vi "Tester.vi"   [LabVIEW 2012]
uses:
  <vilib>/Utility/config.llb/NI_LVConfig.lvlib
  <vilib>/Utility/config.llb/Read Key (Boolean).vi
  <vilib>/Utility/config.llb/Write Key (Boolean).vi
  configlib.lvlib
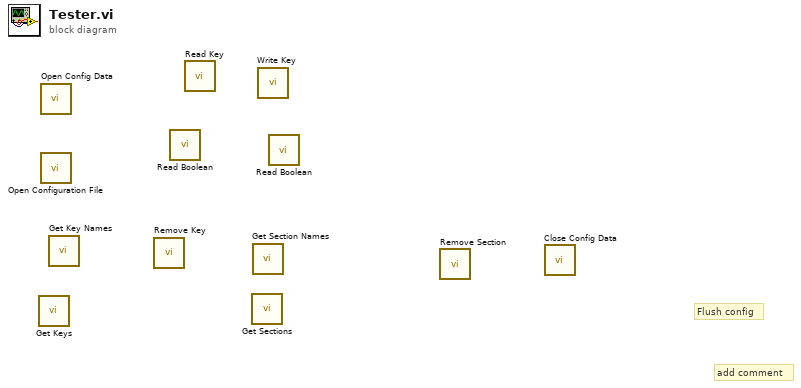
[diagram p0: block diagram]
diagram:
  # "add comment"
  # "Flush config"
  n1 = call "Get Keys.vi"() -> ()  [unwired: 8 in, 4 out]
  n2 = call <vilib>:"Open Config Data.vi"() -> ()  [unwired: 9 in, 3 out]
  n3 = call "Open Configuration File.vi"() -> ()  [unwired: 9 in, 3 out]
  n4 = call <vilib>:"Get Key Names.vi"() -> ()  [unwired: 8 in, 4 out]
  n5 = call <vilib>:"Remove Key.vi"() -> ()  [unwired: 9 in, 3 out]
  n6 = call "Read Boolean.vi"() -> ()  [unwired: 8 in, 4 out]
  n7 = call-poly <vilib>:"Read Key.vi"() -> ()  [unwired: 8 in, 4 out]
  n8 = call "Get Sections.vi"() -> ()  [unwired: 9 in, 3 out]
  n9 = call <vilib>:"Get Section Names.vi"() -> ()  [unwired: 9 in, 3 out]
  n10 = call-poly <vilib>:"Write Key.vi"() -> ()  [unwired: 9 in, 3 out]
  n11 = call "Read Boolean.vi"() -> ()  [unwired: 8 in, 4 out]
  n12 = call <vilib>:"Remove Section.vi"() -> ()  [unwired: 9 in, 3 out]
  n13 = call <vilib>:"Close Config Data.vi"() -> ()  [unwired: 10 in, 2 out]
